vi "Determine Warnings.vi"(8 "error in (no error)":errorcluster, 9 "Min Temp":dbl, 10 "Max Temp":dbl, 11 "Current Temp":dbl) -> (0 "error out":errorcluster, 1 "Warning?":bool, 2 "Warning Text":string)   [LabVIEW 2010]
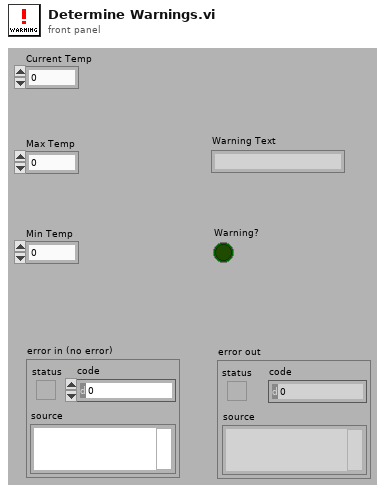
[diagram p1: front panel]
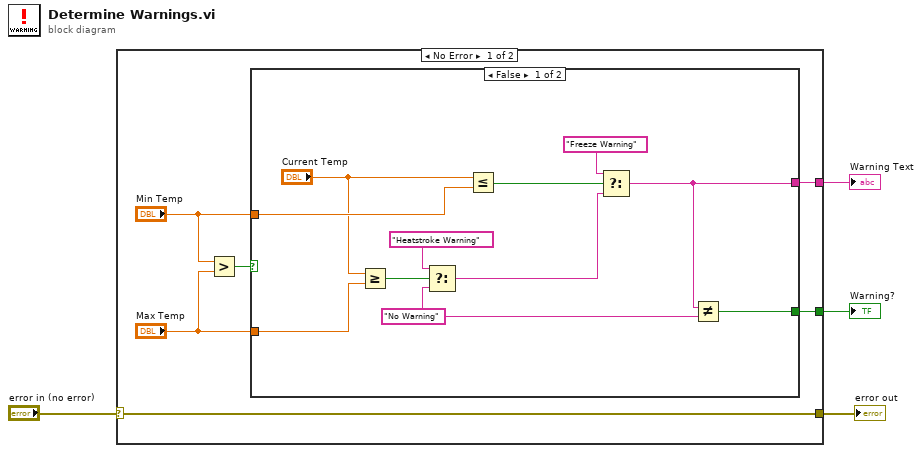
[diagram p0: block diagram]
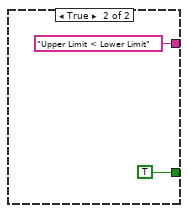
[diagram p2: hidden frame]
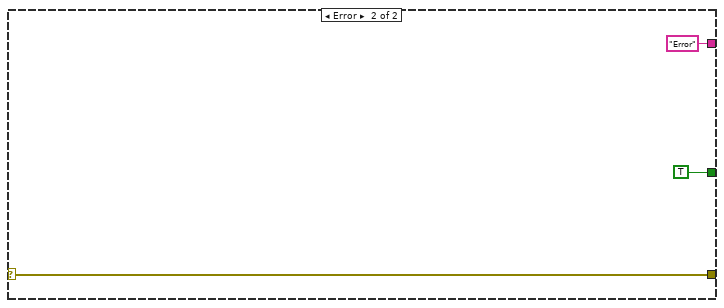
[diagram p3: hidden frame]
diagram:
  n1 = case shown="No Error" "error in (no error)" {
    selector: "error in (no error)" -> [w5 w26]
    tunnel: [w10 "Error" ("f")] -> w4
    tunnel: [w9 TRUE] -> w3
    tunnel: [w5 w26] -> w1
    frame No Error {
      n2 = Greater?(x="Min Temp", y="Max Temp") -> (0:w8:bool)
      n3 = case shown="False" w8 {
        tunnel: [w21 "Upper Limit < Lower Limit" ("f")] -> w10
        tunnel: [w20 TRUE] -> w9
        tunnel: "Max Temp" -> [w19 _]
        tunnel: "Min Temp" -> [w16 _]
        frame False {
          w11 = "No Warning" ("f")
          n4 = Greater Or Equal?(x="Current Temp", y=w19) -> (x >= y?=w18:bool)
          n5 = Select(t="Heatstroke Warning", s=w18, f=w11) -> (s? t:f=w12:string)
          n6 = Less Or Equal?(x="Current Temp", y=w16) -> (x <= y?=w13:bool)
          n7 = Select(t="Freeze Warning", s=w13, f=w12) -> (s? t:f=w21:string)
          n8 = Not Equal?(x=w21, y=w11) -> (x != y?=w20:bool)
        }
        frame True {
        }
      }
    }
    frame Error {
    }
  }
  "Warning Text" <- w4
  "Warning?" <- w3
  "error out" <- w1
